vi "Read Math Measurement.vi"(0 "VISA resource name":refnum<visa-resource-name>, 11 "error in (no error)":errorcluster) -> (4 "VISA resource name out":refnum<visa-resource-name>, 6 "Math Measurements":cluster{dbl[], dbl[]}(graph), 15 "error out":errorcluster)   [LabVIEW 2020, in "Keithley 648X Series.lvlib"]
doc: "Initiates the instrument and reads the fresh math readings.\n\n<b>Note:</b>\nCall the <b>Configure Math Reading VI</b> first, or error \"-230, Data corrupt or stale\" would appear."
uses:
  <instrlib>/Keithley 648X Series/Keithley 648X Series.lvlib
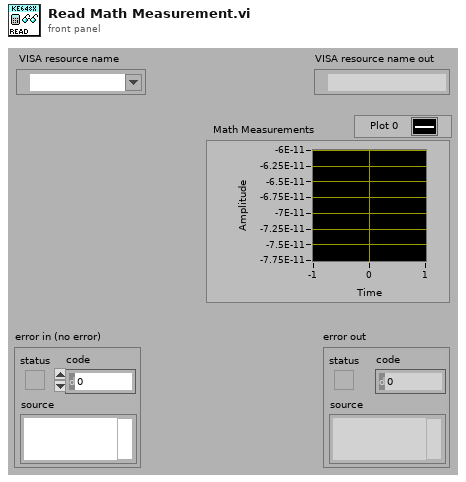
[diagram p1: front panel]
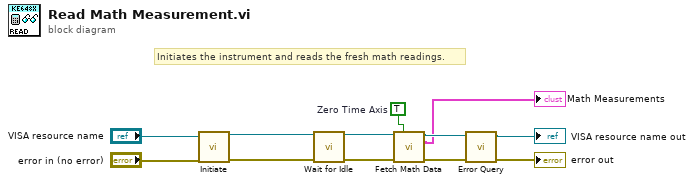
[diagram p0: block diagram]
diagram:
  w1 = TRUE  # Zero Time Axis
  # "Initiates the instrument and reads the fresh math readings."
  n1 = call <instrlib>:"Initiate.vi"("VISA resource name"="VISA resource name", "error in (no error)"="error in (no error)") -> ("VISA resource name out"=w2:refnum<visa-resource-name>, "error out"=w3:errorcluster)  [unwired: 12 in]
  n2 = call <instrlib>:"Wait for Idle.vi"("VISA resource name"=w2, "error in (no error)"=w3) -> ("VISA resource name out"=w6:refnum<visa-resource-name>, "error out"=w7:errorcluster)  [unwired: 12 in]
  n3 = call <instrlib>:"Fetch Math Data.vi"("VISA resource name"=w6, "Zero Time Axis (T)"=w1, "error in (no error)"=w7) -> ("VISA resource name out"=w5:refnum<visa-resource-name>, "Math Data"=→"Math Measurements":cluster{dbl[], dbl[]}, "error out"=w8:errorcluster)  [unwired: 10 in]
  n4 = call <instrlib>:"Error Query.vi"("error in (no error)"=w8, "VISA resource name"=w5) -> ("error out"=→"error out":errorcluster, "VISA resource name out"=→"VISA resource name out":refnum<visa-resource-name>)  [unwired: 6 in, 2 out]
